vi "reql_item_insert.vi"(6 "ms timeout (0:default)":i32, 7 "db name":string, 8 "error in (no error)":errorcluster, 9 "object":variant, 10 "table name":string, 11 "rethinkdb in":refnum<class "RethinkDB.lvclass">) -> (0 "error out":errorcluster, 2 "generated keys":string[](array[string]), 3 "rethinkdb out":refnum<class "RethinkDB.lvclass">, 4 "response":variant)   [LabVIEW 2017, in "rethinkdb.lvlib"]
uses:
  rethinkdb.lvlib
  RethinkDB.lvclass
  ql2_query.ctl
  ql2_term.ctl
  4facdf79-eaab-4117-9226-3fa19dc40407.vi
  json_get_names.vi
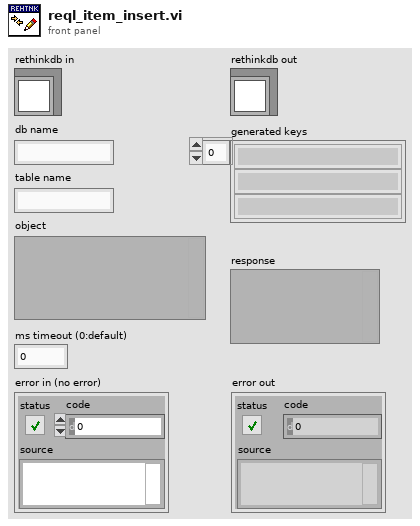
[diagram p1: front panel]
types:
  T1 = typedef "rethinkdb.lvlib/ql2_term.ctl" = enum8{"ADD", "AND", "APPEND", "APRIL", "ARGS", "ASC", "AUGUST", "AVG", "BETWEEN", "BETWEEN_DEPRECATED", "BINARY", "BIT_AND", "BIT_NOT", "BIT_OR", "BIT_SAL", "BIT_SAR", "BIT_XOR", "BRACKET", "BRANCH", "CEIL", "CHANGES", "CHANGE_AT", "CIRCLE", "COERCE_TO", "CONCAT_MAP", "CONFIG", "CONTAINS", "COUNT", "DATE", "DATUM", "DAY", "DAY_OF_WEEK", "DAY_OF_YEAR", "DB", "DB_CREATE", "DB_DROP", "DB_LIST", "DECEMBER", "DEFAULT", "DELETE", "DELETE_AT", "DESC", "DIFFERENCE", "DISTANCE", "DISTINCT", "DIV", "DOWNCASE", "DURING", "EPOCH_TIME", "EQ", "EQ_JOIN", "ERROR", "FEBRUARY", "FILL", "FILTER", "FLOOR", "FOLD", "FOR_EACH", "FRIDAY", "FUNC", "FUNCALL", "GE", "GEOJSON", "GET", "GET_ALL", "GET_FIELD", "GET_INTERSECTING", "GET_NEAREST", "GET_WRITE_HOOK", "GRANT", "GROUP", "GT", "HAS_FIELDS", "HOURS", "HTTP", "IMPLICIT_VAR", "INCLUDES", "INDEX_CREATE", "INDEX_DROP", "INDEX_LIST", "INDEX_RENAME", "INDEX_STATUS", "INDEX_WAIT", "INFO", "INNER_JOIN", "INSERT", "INSERT_AT", "INTERSECTS", "IN_TIMEZONE", "ISO8601", "IS_EMPTY", "JANUARY", "JAVASCRIPT", "JSON", "JULY", "JUNE", "KEYS", "LE", "LIMIT", "LINE", "LITERAL", "LT", "MAKE_ARRAY", "MAKE_OBJ", "MAP", "MARCH", "MATCH", "MAX", "MAXVAL", "MAY", "MERGE", "MIN", "MINUTES", "MINVAL", "MOD", "MONDAY", "MONTH", "MUL", "NE", "NOT", "NOVEMBER", "NOW", "NTH", "OBJECT", "OCTOBER", "OFFSETS_OF", "OR", "ORDER_BY", "OUTER_JOIN", "PLUCK", "POINT", "POLYGON", "POLYGON_SUB", "PREPEND", "RANDOM", "RANGE", "REBALANCE", "RECONFIGURE", "REDUCE", "REPLACE", "ROUND", "SAMPLE", "SATURDAY", "SECONDS", "SEPTEMBER", "SET_DIFFERENCE", "SET_INSERT", "SET_INTERSECTION", "SET_UNION", "SET_WRITE_HOOK", "SKIP", "SLICE", "SPLICE_AT", "SPLIT", "STATUS", "SUB", "SUM", "SUNDAY", "SYNC", "TABLE", "TABLE_CREATE", "TABLE_DROP", "TABLE_LIST", "THURSDAY", "TIME", "TIMEZONE", "TIME_OF_DAY", "TO_EPOCH_TIME", "TO_GEOJSON", "TO_ISO8601", "TO_JSON_STRING", "TUESDAY", "TYPE_OF", "UNGROUP", "UNION", "UPCASE", "UPDATE", "UUID", "VALUES", "VAR", "WAIT", "WEDNESDAY", "WITHOUT", "WITH_FIELDS", "YEAR", "ZIP", "invalid"}
  T2 = typedef "rethinkdb.lvlib/ql2_query.ctl" = enum8{"START", "CONTINUE", "STOP", "NOREPLY_WAIT", "SERVER_INFO", "invalid"}
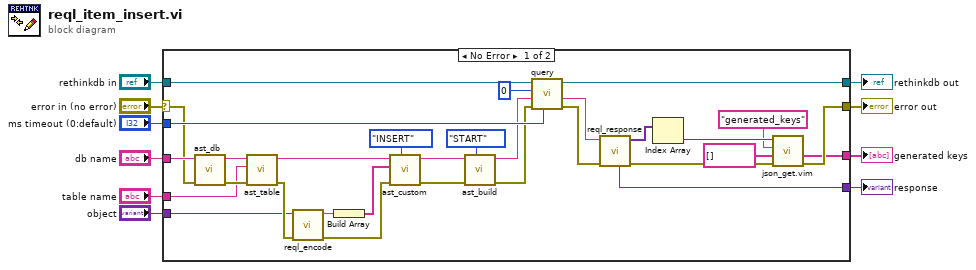
[diagram p0: block diagram]
diagram:
  n1 = case shown="No Error" "error in (no error)" {
    selector: "error in (no error)" -> [w24 w43]
    tunnel: "rethinkdb in" -> [w35 w42]
    tunnel: [w41 w42] -> w8
    tunnel: "ms timeout (0:default)" -> [w40 _]
    tunnel: [w32 w43] -> w6
    tunnel: "db name" -> [w28 _]
    tunnel: "table name" -> [w25 _]
    tunnel: "object" -> [w18 _]
    tunnel: [w30 _] -> w2
    tunnel: [w20 _] -> w1
    frame No Error {
      n2 = call "ast_db.vi"("error in (no error)"=w24, "db name"=w28) -> ("error out"=w26:errorcluster, "r.db"=w27:string)  [unwired: 8 in]
      n3 = call "ast_table.vi"("error in (no error)"=w26, "table name"=w25, "r.db"=w27) -> ("error out"=w19:errorcluster, "r.db.table"=w17:string)  [unwired: 7 in]
      n4 = call "reql_encode.vi"("error in (no error)"=w19, "object"=w18) -> ("error out"=w16:errorcluster, "reql"=w14:string)  [unwired: 8 in]
      n5 = Build Array(w14) -> (w13:string[])
      n6 = call "ast_custom.vi"("term_type"=ql2_term."INSERT", "error in (no error)"=w16, "args"=w13, "arg0"=w17) -> ("error out"=w15:errorcluster, "r"=w12:string)  [unwired: 6 in]
      n7 = call "ast_build.vi"("query_type"=ql2_query."START", "error in (no error)"=w15, "term"=w12) -> ("error out"=w23:errorcluster, "query"=w22:string)  [unwired: 7 in]
      n8 = call "query.vi"("ms timeout (0:default)"=w40, "error in (no error)"=w23, "query"=w22, "token in (random)"=u64 0, "rethinkdb in"=w35) -> ("error out"=w38:errorcluster, "response"=w37:string, "rethinkdb out"=w41:refnum<class "RethinkDB.lvclass">)  [unwired: 3 in, 1 out]
      n9 = call "reql_response.vi"("error in (no error)"=w38, "response"=w37) -> ("error out"=w34:errorcluster, "values"=w36:variant[], "response"=w20:variant)  [unwired: 7 in]
      n10 = Index Array(array=w36) -> (element=w33:variant)  [unwired: 1 in]
      n11 = call "json_get.vim"("error in (no error)"=w34, "default"=string[] [], "name"="generated_keys", "variant in"=w33) -> ("error out"=w32:errorcluster, "value"=w30:string[])  [unwired: 4 in, 2 out]
    }
    frame Error {
    }
  }
  "error out" <- w6
  "rethinkdb out" <- w8
  "response" <- w1
  "generated keys" <- w2
